vi "test_benchmark_search.vi"() -> ()   [LabVIEW 2015]
uses:
  _SubVIs/Advanced/search-double.vi
  binary_search.lvlib
panel:
  out "Error?":bool
  out "Time to Execute (s)":dbl
  in  "Passes":i32=10000
  in  "Elements to Generate":i32=100000
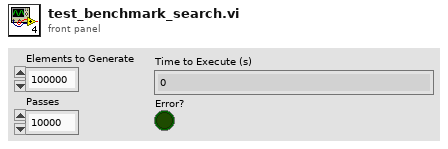
[diagram p1: front panel]
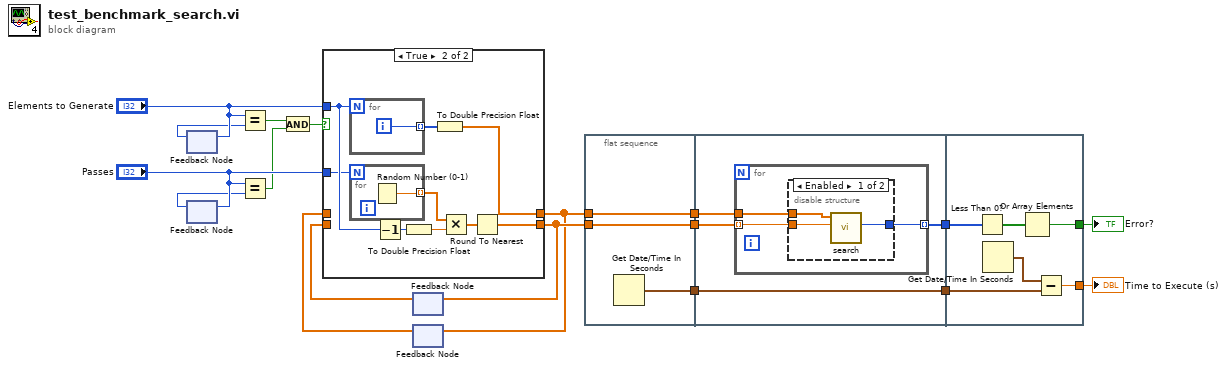
[diagram p0: block diagram]
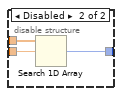
[diagram p3: hidden frame]
diagram:
  n1 = feedback-in #1("Elements to Generate") -> ()
  n2 = feedback #1() -> (w10:i32)  [unwired: 1 in]
  n3 = feedback #2() -> (w8:i32)  [unwired: 1 in]
  n4 = feedback-in #2("Passes") -> ()
  n5 = Equal?(x="Elements to Generate", y=w10) -> (x = y?=w5:bool)
  n6 = Equal?(x="Passes", y=w8) -> (x = y?=w4:bool)
  n7 = And(x=w5, y=w4) -> (x .and. y?=w3:bool)
  n8 = feedback #3() -> (w1:dbl[])  [unwired: 1 in]
  n9 = feedback #4() -> (w2:dbl[])  [unwired: 1 in]
  n10 = case shown="True" w3 {
    tunnel: "Elements to Generate" -> [_ w24]
    tunnel: "Passes" -> [_ w23]
    tunnel: [w19 w22] -> w7
    tunnel: [w20 w21] -> w6
    tunnel: w2 -> [w20 _]
    tunnel: w1 -> [w19 _]
    frame False {
    }
    frame True {
      n11 = for {
        N: w24 -> [_]
        tunnel: [w31] -> w29 mode=indexing
        i -> [w31]
      }
      n12 = for {
        N: w23 -> [_]
        tunnel: [w30] -> w28 mode=indexing
        n13 = Random Number (0-1)() -> (number: 0 to 1=w30:dbl)
      }
      n14 = Decrement(x=w24) -> (x-1=w25:i32)
      n15 = To Double Precision Float(number=w25) -> (double precision float=w27:dbl)
      n16 = To Double Precision Float(number=w29) -> (double precision float=w21:dbl[])
      n17 = Multiply(x=w28, y=w27) -> (x*y=w26:dbl[])
      n18 = Round To Nearest(number=w26) -> (nearest integer value=w22:dbl[])
    }
  }
  n19 = feedback-in #3(w7) -> ()
  n20 = feedback-in #4(w6) -> ()
  n21 = flat-sequence {
    tunnel: w7 -> [w33]
    tunnel: w6 -> [w34]
    tunnel: [w34] -> w18
    tunnel: [w33] -> w17
    tunnel: [w32] -> w16
    tunnel: w18 -> [w38]
    tunnel: w17 -> [w37]
    tunnel: w16 -> [w36]
    tunnel: [w36] -> w15
    tunnel: [w35] -> w13
    tunnel: w15 -> [w52]
    tunnel: [w51] -> w14
    tunnel: w13 -> [w50]
    tunnel: [w48] -> w12
    frame #0 {
      n22 = Get Date/Time In Seconds() -> (seconds since 1Jan1904=w32:timestamp)
    }
    frame #1 {
      n23 = for {
        tunnel: w38 -> [w41]
        tunnel: w37 -> [w40] mode=indexing
        tunnel: [w39] -> w35 mode=indexing
        n24 = disable-structure shown="Enabled" {
          disable-tunnel: w41 -> [w44 w47]
          disable-tunnel: w40 -> [w43 w46]
          disable-tunnel: [w42 w45] -> w39
          frame Enabled {
            n25 = call-poly "search.vi"("Search"=w43, "Data (dbl) []"=w44) -> ("Index"=w42:i32)  [unwired: 9 in]
          }
          frame Disabled {
            n26 = Search 1D Array(1D array=w47, element=w46) -> (index of element=w45:i32)  [unwired: 1 in]
          }
        }
      }
    }
    frame #2 {
      n27 = Less Than 0?(x=w50) -> (x < 0?=w49:bool[])
      n28 = Get Date/Time In Seconds() -> (seconds since 1Jan1904=w53:timestamp)
      n29 = Or Array Elements(Boolean array=w49) -> (logical OR=w48:bool)
      n30 = Subtract(x=w53, y=w52) -> (x-y=w51:dbl)
    }
  }
  "Time to Execute (s)" <- w14
  "Error?" <- w12
